vi "Simple_sound_light_on.vi"() -> ()   [LabVIEW 2019]
panel:
  out "Boolean":bool
  in  "stop":bool
  out "Waveform Chart":dynamicdata(graph)
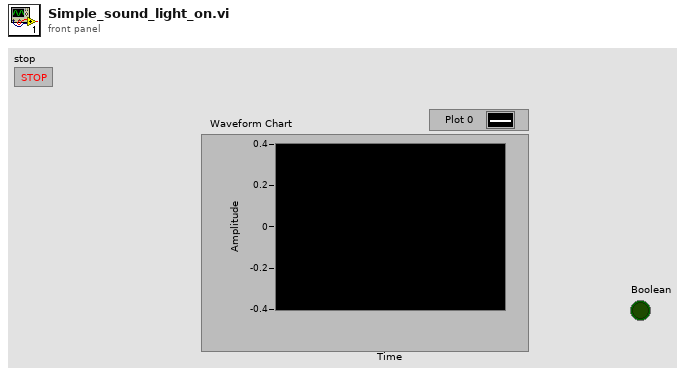
[diagram p1: front panel]
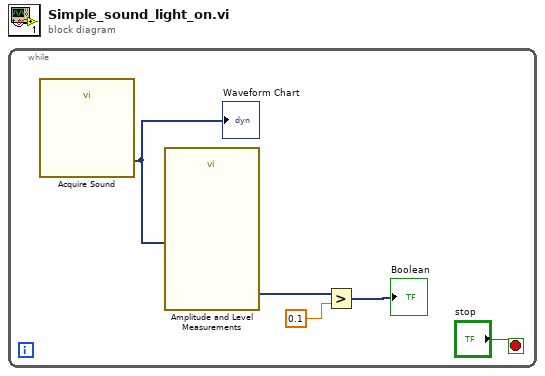
[diagram p0: block diagram]
diagram:
  n1 = while {
    stop <- "stop" stop-if-true
    n2 = call "Acquire Sound"() -> ("Data"=w2:dynamicdata)  [unwired: 18 in, 1 out]
    "Waveform Chart" <- w2
    n3 = call "Amplitude and Level Measurements"("Signals"=w2) -> ("Positive Peak"=w1:dynamicdata)  [unwired: 13 in, 1 out]
    n4 = Greater?(x=w1, y=0.1) -> (0:→"Boolean":dynamicdata)
  }
